vi "主VI.vi"() -> ()   [LabVIEW 2016]
panel:
  in  "确定按钮":bool
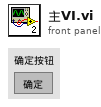
[diagram p1: front panel]
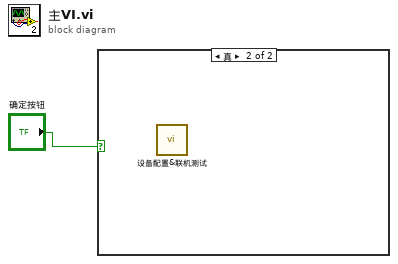
[diagram p0: block diagram]
diagram:
  n1 = case shown="真" "确定按钮" {
    frame False {
    }
    frame True {
      n2 = call "设备配置&联机测试.vi"() -> ()  [unwired: 11 in, 1 out]
    }
  }
